vi "JKI Python Bridge - VI Tree.vi"   [LabVIEW 2020]
uses:
  Server/Server.lvclass
  Call/Call.lvclass
  Server/Register for Events (Single PyObject).vi
  Server/Register for Events (Multiple PyObjects).vi
  Server/Type Definitions/Python Method.ctl
  Server/Type Definitions/Python Object and Method Names - Cluster.ctl
  febeb587-4d39-4063-98b6-da0ee15fd81b.vi
  Server/Register for Events (Multiple PyObjects by Enum).vi
  9c85d652-7377-469b-b200-a7823445b883.vi
types:
  T1 = typedef "jki_python_bridge.lvlib/Server.lvclass/Python Method.ctl" = cluster{"Name":string, "Arguments":string[], "Documentation":string}
  T2 = typedef "jki_python_bridge.lvlib/Server.lvclass/Python Object and Method Names - Cluster.ctl" = cluster{"PyObject Name":string, "Functions":T1[]}
  T3 = enum16{"<unknown python call>", "Object1.HelloWorld", "Object2.Echo", "Object3.Add"}
  T4 = typedef "jki_python_bridge.lvlib/Server.lvclass/Python Method Call - Event Registration.ctl" = refnum<event-registration>
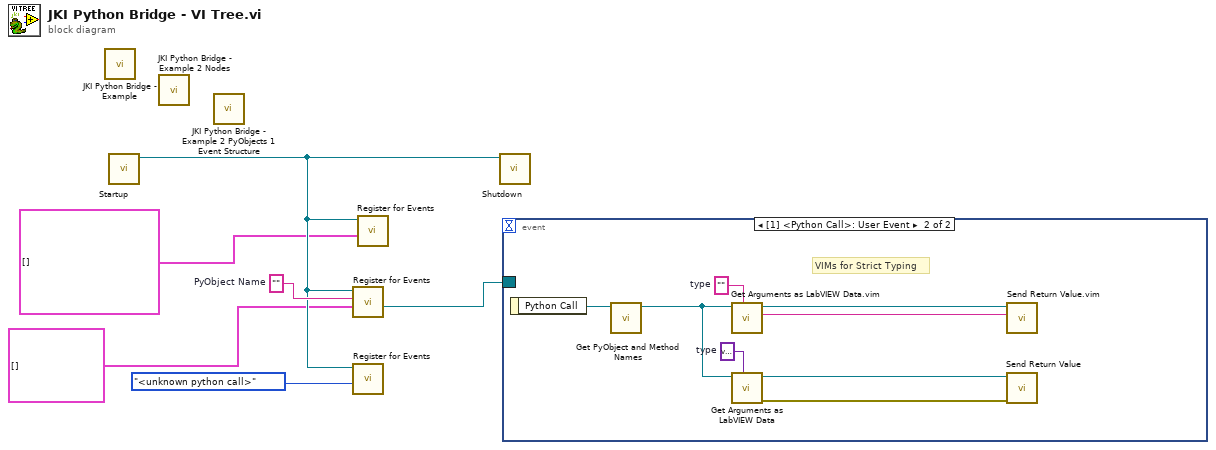
[diagram p0: block diagram]
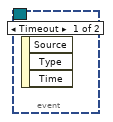
[diagram p2: hidden frame]
diagram:
  w5 = ""  # PyObject Name
  n1 = call "JKI Python Bridge - Example.vi"() -> ()  [unwired: 12 in]
  n2 = call "Startup.vi"() -> ("JKI_Python_Server out"=w4:refnum<class "Server.lvclass">)  [unwired: 10 in, 1 out]
  n3 = call "JKI Python Bridge - Example 2 Nodes.vi"() -> ()  [unwired: 12 in]
  n4 = call "JKI Python Bridge - Example 2 PyObjects 1 Event Structure.vi"() -> ()  [unwired: 12 in]
  n5 = call-poly "Register for Events.vi"("Functions"=T1[] [], "PyObject Name"=w5, "JKI_Python_Server in"=w4) -> ("Python"=w6:T4)  [unwired: 6 in, 2 out]
  n6 = call-poly "Register for Events.vi"("Variant"=T3."<unknown python call>", "JKI_Python_Server in"=w4) -> ()  [unwired: 7 in, 3 out]
  n7 = call-poly "Register for Events.vi"("PyObjects"=T2[] [], "JKI_Python_Server in"=w4) -> ()  [unwired: 7 in, 3 out]
  n8 = call "Shutdown.vi"("JKI_Python_Server in"=w4) -> ()  [unwired: 10 in, 1 out]
  n9 = event shown="[1] <Python Call>: User Event" {
    selector: w6 -> [_ _]
    dyn-events: _ -> [_ _]
    timeout: _ -> [_ _]
    event Timeout {
      n10 = event-data() -> ()  [unwired: 1 in, 3 out]
    }
    event User Event {
      w7 = variant  # type
      w12 = ""  # type
      # "VIMs for Strict Typing"
      n11 = event-data() -> ("Python Call"=w14:refnum<class "Call.lvclass">)  [unwired: 1 in]
      n12 = call "Get PyObject and Method Names.vi"("Call in"=w14) -> ("Call out"=w10:refnum<class "Call.lvclass">)  [unwired: 6 in, 4 out]
      n13 = call "Get Arguments as LabVIEW Data.vim"("type"=w12, "Call in"=w10) -> ("LabVIEW Data"=w11:string, "Call out"=w13:refnum<class "Call.lvclass">)  [unwired: 7 in, 1 out]
      n14 = call "Get Arguments as LabVIEW Data.vi"("type"=w7, "Call in"=w10) -> ("error out"=w8:errorcluster, "Call out"=w9:refnum<class "Call.lvclass">)  [unwired: 7 in, 1 out]
      n15 = call "Send Return Value.vim"("Return Value"=w11, "Response in"=w13) -> ()  [unwired: 9 in, 1 out]
      n16 = call "Send Return Value.vi"("error in (no error)"=w8, "Call in"=w9) -> ()  [unwired: 9 in, 1 out]
    }
  }
